vi "OperationCall.vi"(0 "Add in":refnum<class "Add.lvclass">, 5 "Sub Panel":refnum<vi>, 7 "user event out":refnum<user-event>, 9 "event source":refnum<user-event>, 11 "error in (no error)":errorcluster) -> (4 "Add out":refnum<class "Add.lvclass">, 15 "error out":errorcluster)   [LabVIEW 2023, in "Add.lvclass"]
uses:
  Add.lvclass
  C:/Users/santharu.subramanian/Documents/LV New Assignments/DVR in OOPS/Classes/Arithmetic/Arithmetic.lvclass
  Arithmetic/Arithmetic.lvclass
  AdditionUI.vi
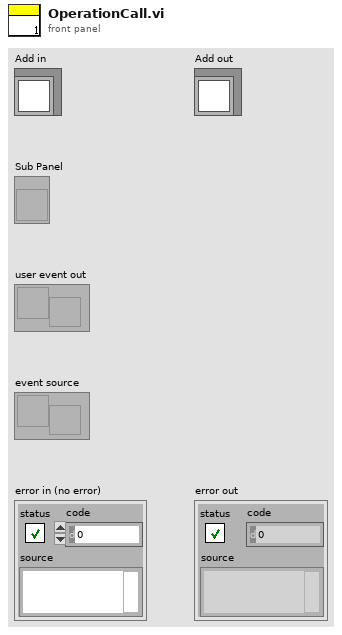
[diagram p1: front panel]
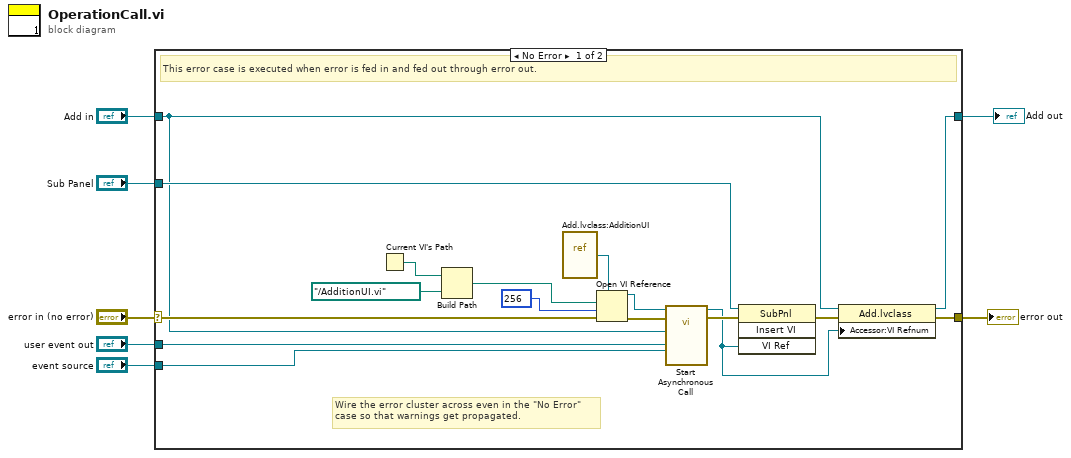
[diagram p0: block diagram]
diagram:
  n1 = case shown="No Error" "error in (no error)" {
    selector: "error in (no error)" -> [w17 w26]
    tunnel: [w11 w26] -> w6
    tunnel: [w10 w25] -> w4
    tunnel: "Add in" -> [w8 w25]
    tunnel: "user event out" -> [w16 _]
    tunnel: "event source" -> [w12 _]
    tunnel: "Sub Panel" -> [w15 _]
    frame No Error {
      # "Wire the error cluster across even in the \"No Error\"\ncase so that warnings get propagated."
      # "This error case is executed when error is fed in and fed out through error out."
      n2 = Current VI's Path() -> (path=w14:path)
      n3 = Build Path(base path=w14, name or relative path=path "../AdditionUI.vi") -> (appended path=w21:path)
      n4 = vi-ref "Add.lvclass:AdditionUI.vi"() -> (w20:refnum<vi>)
      n5 = Open VI Reference(type specifier VI Refnum (for type only)=w20, vi path=w21, options=256, error in (no error)=w17) -> (vi reference=w19:refnum<vi>, error out=w13:errorcluster)  [unwired: 2 in]
      n6 = call-by-ref "Start Asynchronous Call"(reference=w19, error in=w13, "Add in"=w8, "user event out"=w16, "event source"=w12) -> (reference out=w9:refnum<vi>, error out=w23:errorcluster)  [unwired: 10 in, 3 out]
      n7 = invoke on="Invoke Node" class="SubPnl" method="Insert VI"(reference=w15, error in=w23, "VI Ref"=w9) -> (error out=w18:errorcluster)  [unwired: 1 in, 3 out]
      n8 = property class="Add.lvclass"(reference=w8, error in=w18, "Accessor:VI Refnum"=w9) -> (reference out=w10:refnum<class "Add.lvclass">, error out=w11:errorcluster)
    }
    frame Error {
      # "This error case is executed when error is fed in and fed out through error out."
    }
  }
  "error out" <- w6
  "Add out" <- w4
